vi "calculate sonde parameter cluster.vi"(6 "tolerance limit":dbl, 7 "Cluster in":T1 {"%" format="%_2f%%"; "Value" format="%_4g"}, 8 "error in (no error)":errorcluster, 9 "Read % value":dbl, 10 "Read Value":dbl, 11 "Initial Value":dbl) -> (0 "error out":errorcluster, 1 "Tolerance":bool, 2 "%":dbl, 3 "Cluster Out":T1 {"%" format="%_2f%%"; "Value" format="%_4g"})   [LabVIEW 2016]
uses:
  Sonde Value Percent Tol.ctl
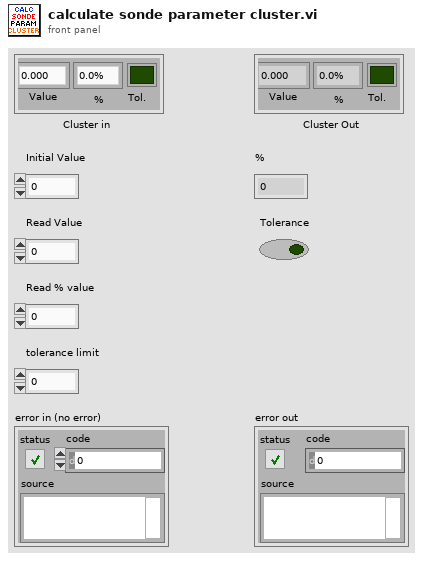
[diagram p1: front panel]
types:
  T1 = typedef "Sonde Value Percent Tol.ctl" = cluster{"Value":dbl, "%":dbl, "Tol.":bool}
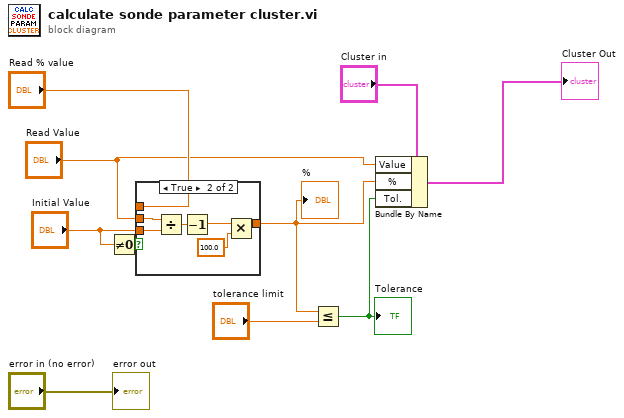
[diagram p0: block diagram]
diagram:
  n1 = Not Equal To 0?(x="Initial Value") -> (x != 0?=w6:bool)
  n2 = case shown="True" w6 {
    tunnel: "Read Value" -> [_ w17]
    tunnel: "Initial Value" -> [_ w16]
    tunnel: [w11 w14] -> w9
    tunnel: "Read % value" -> [w11 _]
    frame False {
    }
    frame True {
      n3 = Divide(x=w17, y=w16) -> (x/y=w15:dbl)
      n4 = Decrement(x=w15) -> (x-1=w12:dbl)
      n5 = Multiply(x=w12, y=100.0) -> (x*y=w14:dbl)
    }
  }
  "%" <- w9
  n6 = Less Or Equal?(x=w9, y="tolerance limit") -> (x <= y?=w3:bool)
  "Tolerance" <- w3
  n7 = Bundle By Name(cluster="Cluster in", "Value"="Read Value", "%"=w9, "Tol."=w3) -> (→"Cluster Out":T1)
  "error out" <- "error in (no error)"
